vi "MindwaveParseData.vi"(1 "RAW_ARRAY":u8[](array[numeric]) format="%x", 2 "canParseData?":bool) -> (0 "MindWave":T1)   [LabVIEW 2011, in "Neurosky.lvlib"]
doc: "Parse values of \nEEG_POWER\nPOOR_QUALITY\ndelta wave"
uses:
  Users/Isaias/Documents/GitHub/Neurosky/Neurosky.lvlib
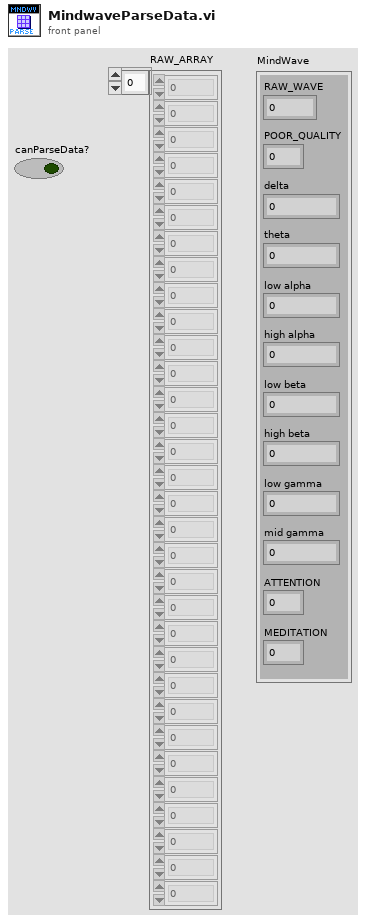
[diagram p1: front panel]
types:
  T1 = cluster{"RAW_WAVE":i16, "POOR_QUALITY":u8, "delta":sgl, "theta":sgl, "low alpha":sgl, "high alpha":sgl, "low beta":sgl, "high beta":sgl, "low gamma":sgl, "mid gamma":sgl, "ATTENTION":u8, "MEDITATION":u8}
  T2 = cluster{"[0]":u32, "[1]":u32, "[2]":u32, "[3]":u32, "[4]":u32, "[5]":u32, "[6]":u32, "[7]":u32, "[8]":u32}
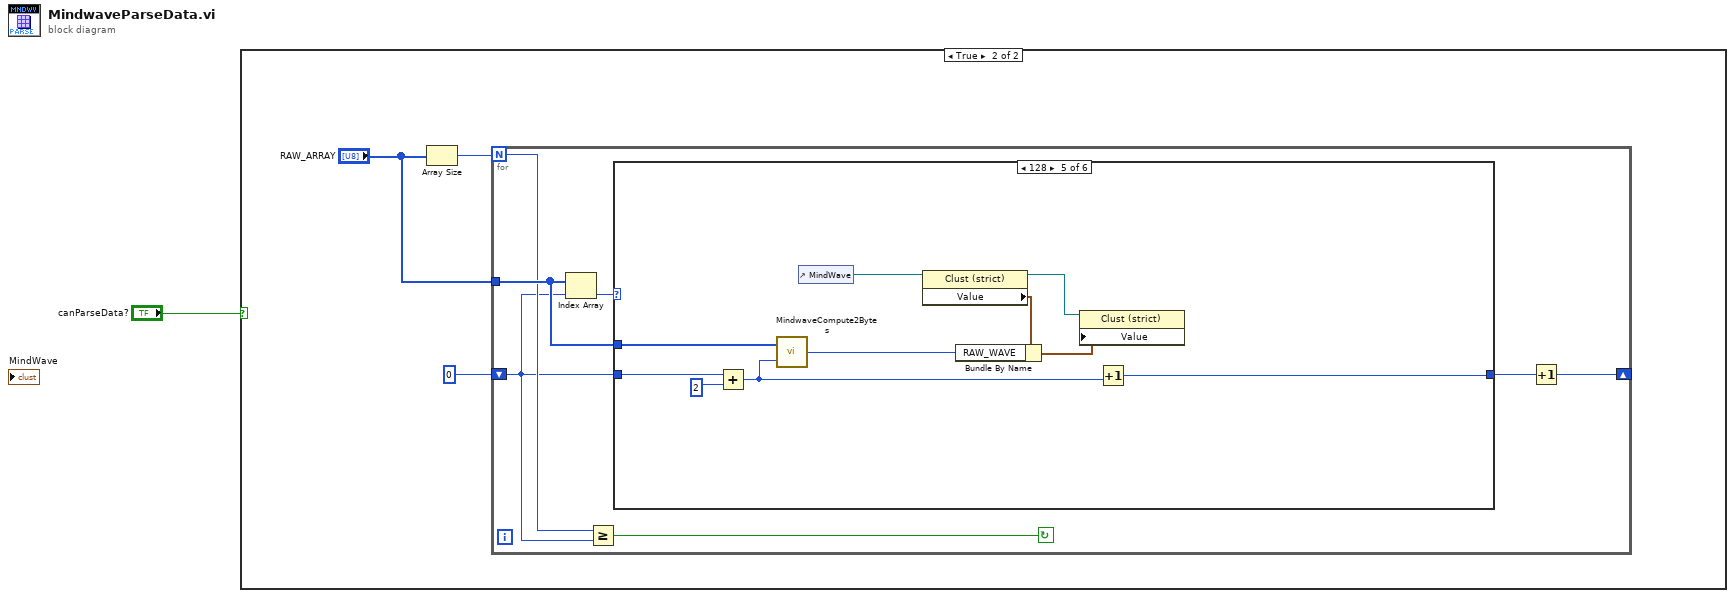
[diagram p0: block diagram]
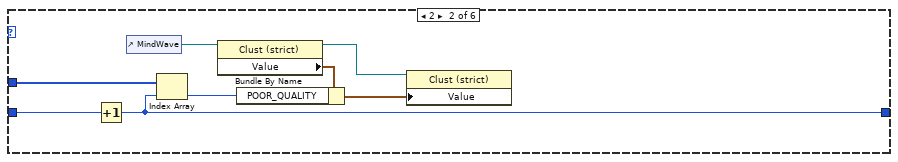
[diagram p4: hidden frame]
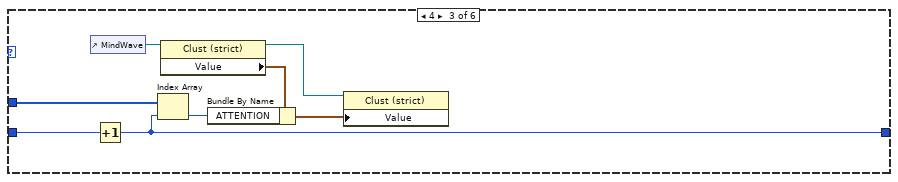
[diagram p5: hidden frame]
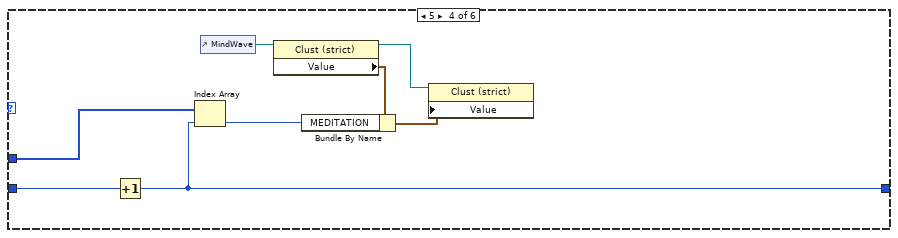
[diagram p6: hidden frame]
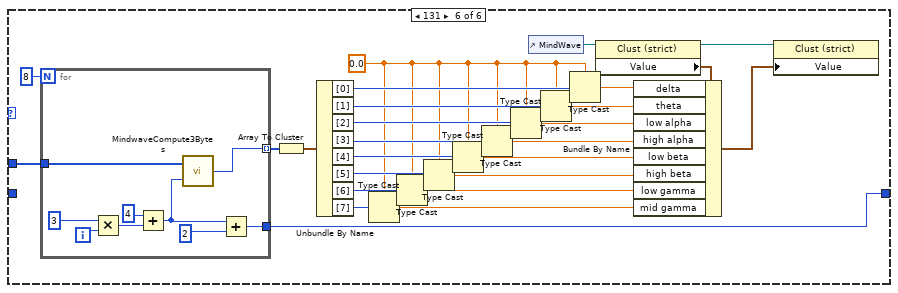
[diagram p7: hidden frame]
diagram:
  n1 = case shown="True" "canParseData?" {
    frame False {
    }
    frame True {
      n2 = Array Size(array="RAW_ARRAY") -> (size(s)=w4:i32)
      n3 = for {
        N: w4 -> [w8]
        tunnel: "RAW_ARRAY" -> [w10]
        shift-right: [w6] -> _
        shift-left: 0 -> [w7]
        stop <- w9 continue-if-true
        n4 = Index Array(array=w10, index=w7) -> (element=w11:u8)
        n5 = Greater Or Equal?(x=w8, y=w7) -> (x >= y?=w9:bool)
        n6 = case shown="128" w11 {
          tunnel: w7 -> [w12 w20 w28 w35 w44 _]
          tunnel: [w12 w13 w21 w34 w38 w64] -> w5
          tunnel: w10 -> [_ w19 w27 w36 w46 w72]
          frame 0, Default {
          }
          frame 2 {
            n7 = Increment(x=w20) -> (x+1=w13:i32)
            n8 = control-ref of="MindWave"() -> (w15:refnum<vi>)
            n9 = Index Array(array=w19, index=w13) -> (element=w14:u8)
            n10 = property on="Property Node" class="Clust (strict)"(reference=w15) -> (reference out=w17:refnum<vi>, "Value"=w16:T1)  [unwired: 1 in, 1 out]
            n11 = Bundle By Name(cluster=w16, "POOR_QUALITY"=w14) -> (w18:T1)
            n12 = property on="Property Node" class="Clust (strict)"(reference=w17, "Value"=w18) -> ()  [unwired: 1 in, 2 out]
          }
          frame 4 {
            n13 = control-ref of="MindWave"() -> (w22:refnum<vi>)
            n14 = Increment(x=w28) -> (x+1=w21:i32)
            n15 = Index Array(array=w27, index=w21) -> (element=w23:u8)
            n16 = property on="Property Node" class="Clust (strict)"(reference=w22) -> (reference out=w25:refnum<vi>, "Value"=w24:T1)  [unwired: 1 in, 1 out]
            n17 = Bundle By Name(cluster=w24, "ATTENTION"=w23) -> (w26:T1)
            n18 = property on="Property Node" class="Clust (strict)"(reference=w25, "Value"=w26) -> ()  [unwired: 1 in, 2 out]
          }
          frame 5 {
            n19 = Increment(x=w35) -> (x+1=w34:i32)
            n20 = Index Array(array=w36, index=w34) -> (element=w29:u8)
            n21 = control-ref of="MindWave"() -> (w30:refnum<vi>)
            n22 = property on="Property Node" class="Clust (strict)"(reference=w30) -> (reference out=w32:refnum<vi>, "Value"=w33:T1)  [unwired: 1 in, 1 out]
            n23 = Bundle By Name(cluster=w33, "MEDITATION"=w29) -> (w31:T1)
            n24 = property on="Property Node" class="Clust (strict)"(reference=w32, "Value"=w31) -> ()  [unwired: 1 in, 2 out]
          }
          frame 128 {
            n25 = Add(x=w44, y=2) -> (x+y=w37:i32)
            n26 = call <userlib>:"MindwaveCompute2Bytes.vi"("INDEX"=w37, "RAW_ARRAY"=w46) -> ("RAW_VALUE"=w39:i16)
            n27 = control-ref of="MindWave"() -> (w40:refnum<vi>)
            n28 = property on="Property Node" class="Clust (strict)"(reference=w40) -> (reference out=w42:refnum<vi>, "Value"=w43:T1)  [unwired: 1 in, 1 out]
            n29 = Bundle By Name(cluster=w43, "RAW_WAVE"=w39) -> (w41:T1)
            n30 = property on="Property Node" class="Clust (strict)"(reference=w42, "Value"=w41) -> ()  [unwired: 1 in, 2 out]
            n31 = Increment(x=w37) -> (x+1=w38:i32)
          }
          frame 131 {
            w47 = sgl 0.0
            n32 = for {
              N: 8 -> [_]
              tunnel: w72 -> [w73]
              tunnel: [w78] -> w66 mode=indexing
              tunnel: [w74] -> w64
              i -> [w81]
              n33 = Multiply(x=3, y=w81) -> (x*y=w77:i32)
              n34 = Add(x=4, y=w77) -> (x+y=w76:i32)
              n35 = call <userlib>:"MindwaveCompute3Bytes.vi"("INDEX"=w76, "RAW_ARRAY"=w73) -> ("RAW_VALUE"=w78:u32)
              n36 = Add(x=w76, y=2 ("x")) -> (x+y=w74:i32)
            }
            n37 = Array To Cluster(array=w66) -> (cluster=w65:T2)
            n38 = Unbundle By Name(w65) -> ("[0]"=w63:u32, "[1]"=w60:u32, "[2]"=w58:u32, "[3]"=w56:u32, "[4]"=w54:u32, "[5]"=w52:u32, "[6]"=w50:u32, "[7]"=w48:u32)
            n39 = Type Cast(type=w47, x=w48) -> (*(type *) &x=w49:sgl)
            n40 = Type Cast(type=w47, x=w50) -> (*(type *) &x=w51:sgl)
            n41 = Type Cast(type=w47, x=w52) -> (*(type *) &x=w53:sgl)
            n42 = Type Cast(type=w47, x=w54) -> (*(type *) &x=w55:sgl)
            n43 = Type Cast(type=w47, x=w56) -> (*(type *) &x=w57:sgl)
            n44 = Type Cast(type=w47, x=w58) -> (*(type *) &x=w59:sgl)
            n45 = control-ref of="MindWave"() -> (w70:refnum<vi>)
            n46 = Type Cast(type=w47, x=w60) -> (*(type *) &x=w61:sgl)
            n47 = Type Cast(type=w47, x=w63) -> (*(type *) &x=w62:sgl)
            n48 = property on="Property Node" class="Clust (strict)"(reference=w70) -> (reference out=w68:refnum<vi>, "Value"=w67:T1)  [unwired: 1 in, 1 out]
            n49 = Bundle By Name(cluster=w67, "delta"=w62, "theta"=w61, "low alpha"=w59, "high alpha"=w57, "low beta"=w55, "high beta"=w53, "low gamma"=w51, "mid gamma"=w49) -> (w69:T1)
            n50 = property on="Property Node" class="Clust (strict)"(reference=w68, "Value"=w69) -> ()  [unwired: 1 in, 2 out]
          }
        }
        n51 = Increment(x=w5) -> (x+1=w6:i32)
      }
    }
  }
